vi "Read endstops.vi"(8 "error in (no error)":errorcluster, 10 "Ens-stop state in":bool[](array[boolean])=[FALSE, FALSE], 11 "VISA Refnum in":refnum<visa-resource-name>) -> (0 "error out":errorcluster, 2 "Ens-stop state":bool[](array[boolean]), 3 "VISA Refnum out":refnum<visa-resource-name>)   [LabVIEW 2020, in "Control de MaP.lvlib"]
uses:
  Control de MaP.lvlib
  Write--command.vi
  <vilib>/Instr/_visa.llb/VISA Flush IO Buffer Mask.ctl
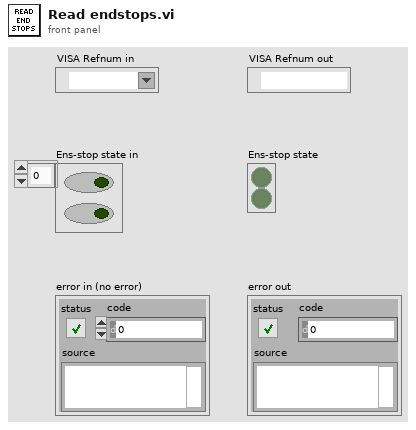
[diagram p1: front panel]
types:
  T1 = typedef "VISA Flush IO Buffer Mask.ctl" = u16
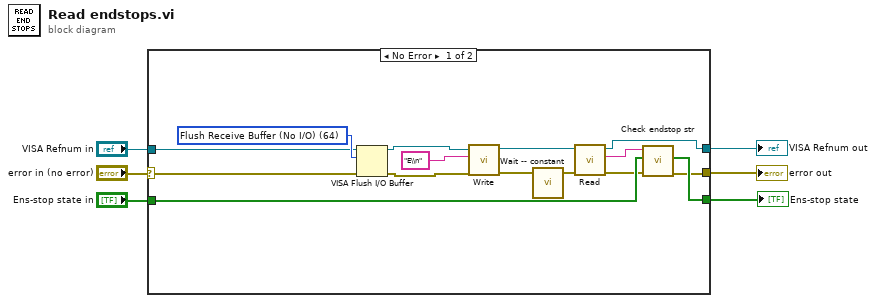
[diagram p0: block diagram]
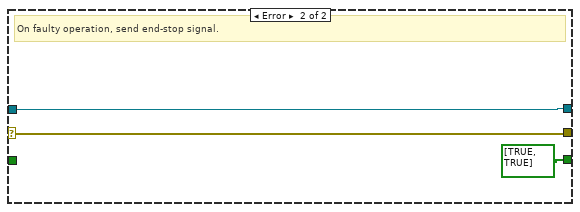
[diagram p2: hidden frame]
diagram:
  n1 = case shown="No Error" "error in (no error)" {
    selector: "error in (no error)" -> [w17 w23]
    tunnel: [w21 bool[] [TRUE, TRUE] ("Ens-stop state out")] -> w6
    tunnel: "VISA Refnum in" -> [w15 w24]
    tunnel: [w13 w24] -> w3
    tunnel: [w7 w23] -> w2
    tunnel: "Ens-stop state in" -> [w9 _]
    frame No Error {
      w19 = T1 64 items=["Flush Receive Buffer"=16, "Write Transmit Buffer to Device"=32, "Flush Receive Buffer (No I/O)"=64, "Flush Transmit Buffer"=128] ("Mask")
      n2 = VISA Flush I/O Buffer(VISA resource name=w15, mask (16)=w19, error in (no error)=w17) -> (VISA resource name out=w16:refnum<visa-resource-name>, error out=w18:errorcluster)
      n3 = call-poly "Write.vi"("error in (no error)"=w18, "Command"="E\\n", "VISA resource name"=w16) -> ("error out"=w10:errorcluster, "VISA resource name out"=w12:refnum<visa-resource-name>)  [unwired: 6 in, 1 out]
      n4 = call "Wait -- constant.vi"("error in (no error)"=w10) -> ("error out"=w11:errorcluster)  [unwired: 4 in]
      n5 = call "Read.vi"("error in (no error)"=w11, "VISA resource name"=w12) -> ("error out"=w8:errorcluster, "Recibo de Datos"=w20:string, "VISA resource name out"=w13:refnum<visa-resource-name>)  [unwired: 6 in, 1 out]
      n6 = call "Check endstop str.vi"("error in (no error)"=w8, "Ens-stop state in"=w9, "Data in"=w20) -> ("error out"=w7:errorcluster, "Ens-stop state out"=w21:bool[])  [unwired: 7 in]
    }
    frame Error {
      # "On faulty operation, send end-stop signal."
    }
  }
  "Ens-stop state" <- w6
  "VISA Refnum out" <- w3
  "error out" <- w2
